vi "Resize UI.vi"(11 "UI Refs In":T1) -> (3 "UI Refs":T1)   [LabVIEW 2020, in "OOPanel.lvlib" / "ArrayManager.lvclass"]
uses:
  ArrayManager.lvclass
  UI Refs.ctl
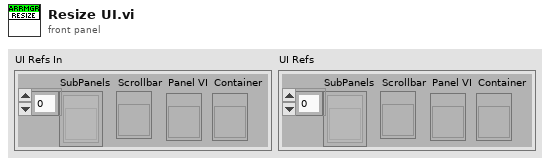
[diagram p1: front panel]
types:
  T1 = typedef "OOPanel.lvlib/ArrayManager.lvclass/UI Refs.ctl" = cluster{"SubPanels":refnum<vi>[], "Scrollbar":refnum<vi>, "Panel VI":refnum<vi>, "Container":refnum<vi>}
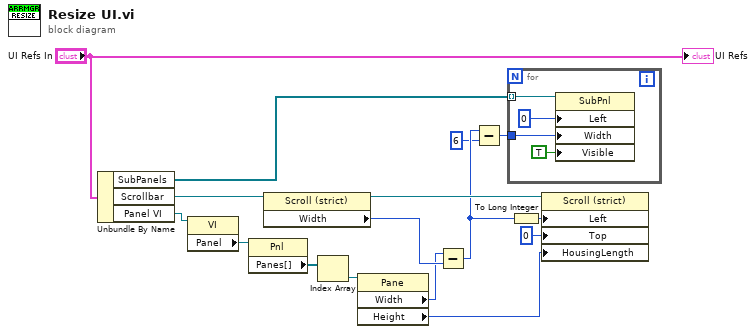
[diagram p0: block diagram]
diagram:
  n1 = Unbundle By Name("UI Refs In") -> ("SubPanels"=w5:refnum<vi>[], "Scrollbar"=w14:refnum<vi>, "Panel VI"=w1:refnum<vi>)
  n2 = property class="VI"(reference=w1) -> ("Panel"=w16:refnum<vi>)  [unwired: 1 in, 2 out]
  n3 = property class="Pnl"(reference=w16) -> ("Panes[]"=w9:refnum<vi>[])  [unwired: 1 in, 2 out]
  n4 = property class="Scroll (strict)"(reference=w14) -> (reference out=w12:refnum<vi>, "Width"=w13:u32)  [unwired: 1 in, 1 out]
  n5 = Index Array(array=w9) -> (element=w8:refnum<vi>)  [unwired: 1 in]
  n6 = property class="Pane"(reference=w8) -> ("Width"=w7:u32, "Height"=w6:u32)  [unwired: 1 in, 2 out]
  n7 = Subtract(x=w7, y=w13) -> (x-y=w4:u32)
  n8 = Subtract(x=w4, y=u32 6) -> (x-y=w3:u32)
  n9 = for {
    tunnel: w5 -> [w20] mode=indexing
    tunnel: w3 -> [w18]
    n10 = property class="SubPnl"(reference=w20, "Left"=0 ("Position:Left"), "Width"=w18, "Visible"=TRUE) -> ()  [unwired: 1 in, 2 out]
  }
  n11 = To Long Integer(number=w4) -> (32bit integer=w11:i32)
  n12 = property class="Scroll (strict)"(reference=w12, "Left"=w11, "Top"=0 ("Position:Top"), "HousingLength"=w6) -> ()  [unwired: 1 in, 2 out]
  "UI Refs" <- "UI Refs In"
